vi "date and time.vi"() -> (4 "date/time string":string, 5 "date/time string 2":string, 6 "date/time string 3":string)   [LabVIEW 2020]
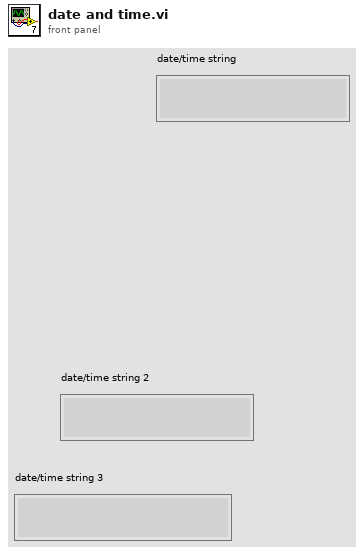
[diagram p1: front panel]
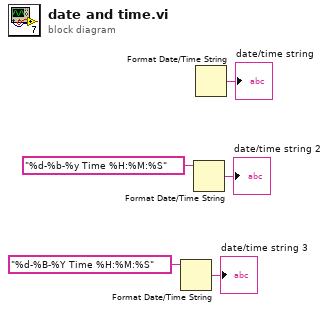
[diagram p0: block diagram]
diagram:
  n1 = Format Date/Time String(time format string (%c)="%d-%B-%Y Time %H:%M:%S") -> (date/time string=→"date/time string 3":string)  [unwired: 2 in]
  n2 = Format Date/Time String(time format string (%c)="%d-%b-%y Time %H:%M:%S") -> (date/time string=→"date/time string 2":string)  [unwired: 2 in]
  n3 = Format Date/Time String() -> (date/time string=→"date/time string":string)  [unwired: 3 in]
